vi "Process1.vi"(8 "error in (no error)":errorcluster, 11 "Object ref in":T1) -> (0 "error out":errorcluster, 3 "Object ref out":T1)   [LabVIEW 2013, in "MaterialCharacterization.lvlib" / "MC-Main.lvclass"]
uses:
  MC-Main.lvclass
  Object-reference.ctl
  Process1-actions.ctl
  Main-actions.ctl
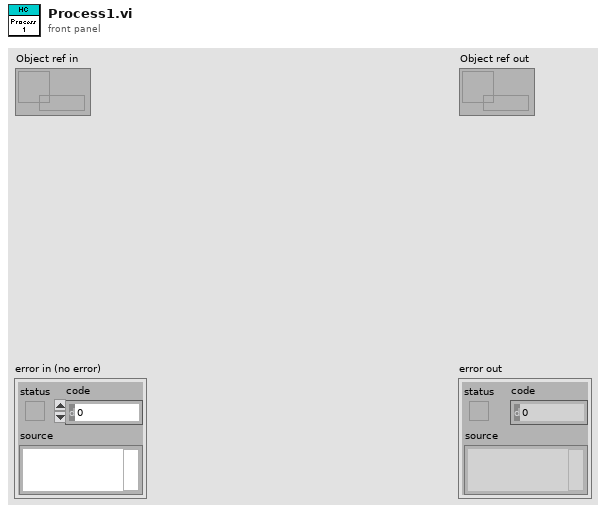
[diagram p1: front panel]
types:
  T1 = typedef "MaterialCharacterization.lvlib/MC-Main.lvclass/Object-reference.ctl" = refnum<data-value>
  T2 = typedef "MaterialCharacterization.lvlib/MC-Main.lvclass/Process1-actions.ctl" = enum16{"Idle", "Activate", "Analyse scan file", "Convert SM1000positions", "Measure SM1000 timings", "Measure laser timings", "Stop", "Abort", "Exit"}
  T3 = typedef "MaterialCharacterization.lvlib/MC-Main.lvclass/Main-actions.ctl" = enum16{"Idle", "Initialize", "Load configuration", "Save configuration", "Load file", "Edit settings", "View scan file", "View raw path", "Edit measurement settings", "Activate", "Start", "Stop", "Refresh display", "Exit"}
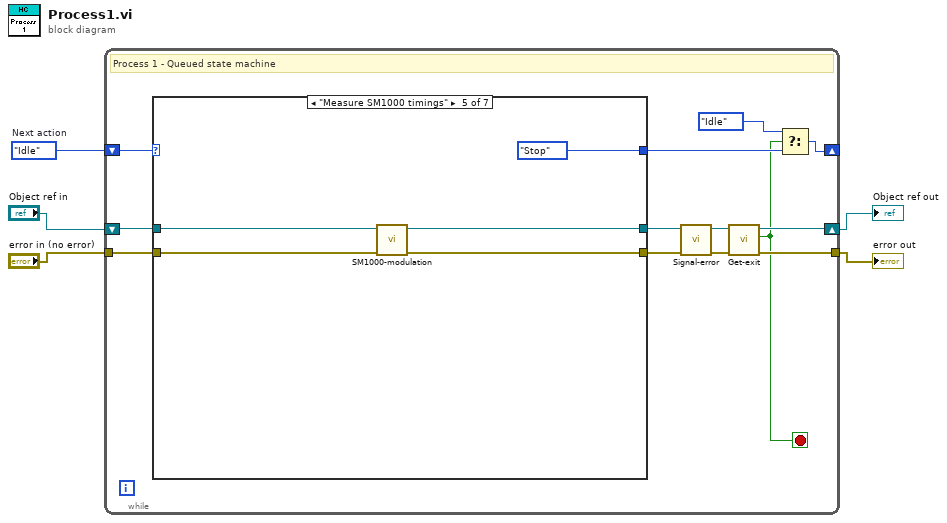
[diagram p0: block diagram]
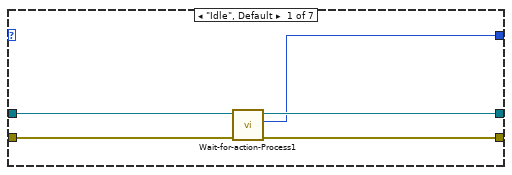
[diagram p2: hidden frame]
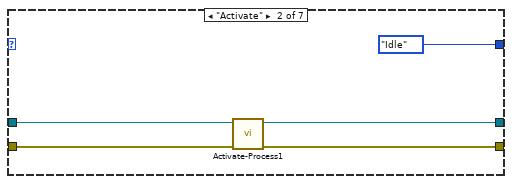
[diagram p3: hidden frame]
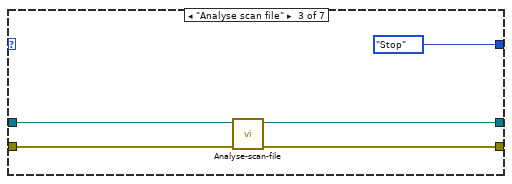
[diagram p4: hidden frame]
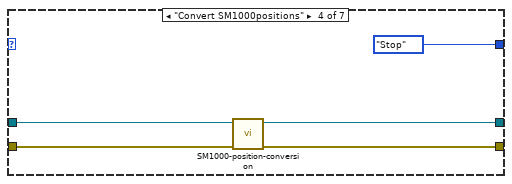
[diagram p5: hidden frame]
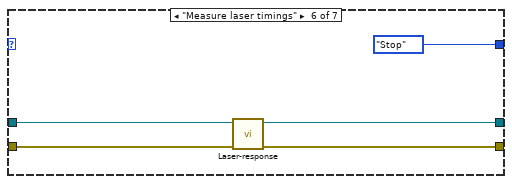
[diagram p6: hidden frame]
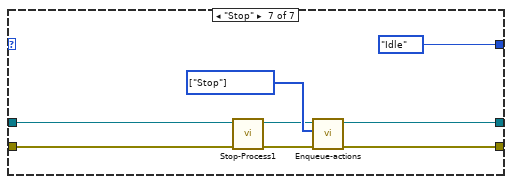
[diagram p7: hidden frame]
diagram:
  w5 = Process1-actions."Idle"  # Next action
  n1 = while {
    shift-right: [w10] -> _
    shift-left: w5 -> [w18]
    shift-right: [w13] -> w3
    shift-left: "Object ref in" -> [w16]
    tunnel: "error in (no error)" -> [w17]
    tunnel: [w8] -> w4
    stop <- w6 stop-if-true
    # "Process 1 - Queued state machine"
    n2 = case shown="\"Measure SM1000 timings\"" w18 {
      tunnel: w17 -> [w19 w25 w30 w35 w40 w45 w50]
      tunnel: [w21 w24 w29 w34 w39 w44 w54] -> w7
      tunnel: [w20 Process1-actions."Idle" ("Action Handler states") Process1-actions."Stop" ("Action Handler states") Process1-actions."Stop" ("Action Handler states") Process1-actions."Stop" ("Action Handler states") Process1-actions."Stop" ("Action Handler states") Process1-actions."Idle" ("Action Handler states")] -> w11
      tunnel: w16 -> [w23 w27 w32 w37 w42 w47 w56]
      tunnel: [w22 w26 w31 w36 w41 w46 w55] -> w15
      frame "Idle", Default {
        n3 = call "Wait-for-action-Process1.vi"("error in (no error)"=w19, "Object ref in"=w23) -> ("error out"=w21:errorcluster, "Action"=w20:T2, "Object ref out"=w22:T1)  [unwired: 7 in]
      }
      frame "Activate" {
        n4 = call "Activate-Process1.vi"("error in (no error)"=w25, "Object ref in"=w27) -> ("error out"=w24:errorcluster, "Object ref out"=w26:T1)  [unwired: 8 in]
      }
      frame "Analyse scan file" {
        n5 = call "Analyse-scan-file.vi"("error in (no error)"=w30, "Object ref in"=w32) -> ("error out"=w29:errorcluster, "Object ref out"=w31:T1)  [unwired: 8 in]
      }
      frame "Convert SM1000positions" {
        n6 = call "SM1000-position-conversion.vi"("error in (no error)"=w35, "Object ref in"=w37) -> ("error out"=w34:errorcluster, "Object ref out"=w36:T1)  [unwired: 8 in]
      }
      frame "Measure SM1000 timings" {
        n7 = call "SM1000-modulation.vi"("error in (no error)"=w40, "Object ref in"=w42) -> ("error out"=w39:errorcluster, "Object ref out"=w41:T1)  [unwired: 8 in]
      }
      frame "Measure laser timings" {
        n8 = call "Laser-response.vi"("error in (no error)"=w45, "Object ref in"=w47) -> ("error out"=w44:errorcluster, "Object ref out"=w46:T1)  [unwired: 8 in]
      }
      frame "Stop" {
        w52 = T3[] [enum."Stop"] items=["Idle", "Initialize", "Load configuration", "Save configuration", "Load file", "Edit settings", "View scan file", "View raw path", "Edit measurement settings", "Activate", "Start", "Stop", "Refresh display", "Exit"] ("State array")
        n9 = call "Stop-Process1.vi"("error in (no error)"=w50, "Object ref in"=w56) -> ("error out"=w49:errorcluster, "Object ref out"=w51:T1)  [unwired: 8 in]
        n10 = call "Enqueue-actions.vi"("error in (no error)"=w49, "State array"=w52, "State queue in"=w51) -> ("error out"=w54:errorcluster, "State queue out"=w55:T1)  [unwired: 6 in, 1 out]
      }
    }
    n11 = call "Signal-error.vi"("error in (no error)"=w7, "Data in"=w15) -> ("error out"=w12:errorcluster, "Data out"=w14:T1)  [unwired: 8 in]
    n12 = call "Get-exit.vi"("error in (no error)"=w12, "Object ref in"=w14) -> ("error out"=w8:errorcluster, "Exit?"=w6:bool, "Object ref out"=w13:T1)  [unwired: 7 in]
    n13 = Select(t=Process1-actions."Idle", s=w6, f=w11) -> (s? t:f=w10:T2)
  }
  "error out" <- w4
  "Object ref out" <- w3
